vi "Graham Scan Dot Product.vi"(1 "B":T1, 2 "A":T1) -> (0 "C":i32)   [LabVIEW 2018]
uses:
  Graham Scan Point.ctl
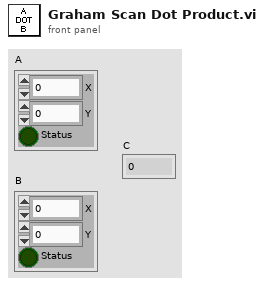
[diagram p1: front panel]
types:
  T1 = typedef "Graham Scan Point.ctl" = cluster{"X":i32, "Y":i32, "Status":bool}
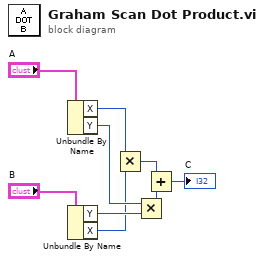
[diagram p0: block diagram]
diagram:
  n1 = Unbundle By Name("A") -> ("X"=w9:i32, "Y"=w6:i32)
  n2 = Unbundle By Name("B") -> ("Y"=w3:i32, "X"=w2:i32)
  n3 = Multiply(x=w9, y=w2) -> (x*y=w8:i32)
  n4 = Multiply(x=w6, y=w3) -> (x*y=w7:i32)
  n5 = Add(x=w8, y=w7) -> (x+y=→"C":i32)
